vi "buttons_disabler.vi"(10 "Array":refnum<vi>[](array[refnum]), 11 "s":bool) -> ()   [LabVIEW 2017]
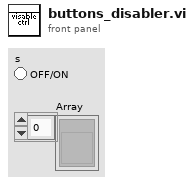
[diagram p1: front panel]
types:
  T1 = enum8{"Enabled", "Disabled", "Disabled and Grayed Out"}
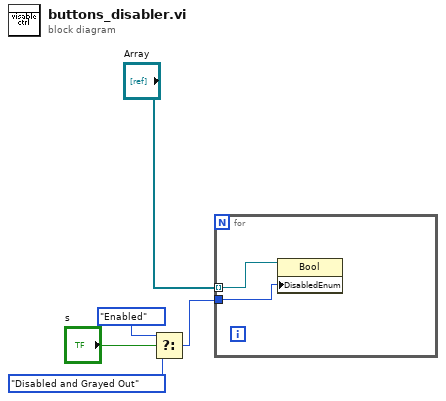
[diagram p0: block diagram]
diagram:
  n1 = Select(t=T1."Enabled" ("Disabled"), s="s", f=T1."Disabled and Grayed Out" ("Disabled")) -> (s? t:f=w5:T1)
  n2 = for {
    tunnel: "Array" -> [w7] mode=indexing
    tunnel: w5 -> [w6]
    n3 = property class="Bool"(reference=w7, "DisabledEnum"=w6) -> ()  [unwired: 1 in, 2 out]
  }
